vi "create_marker_channel.vi"(10 "Data from Stream":cluster{"LED1?":bool, "Data":dbl}[](array[cluster])) -> (1 "LED1?":waveform(dbl), 2 "Signal":waveform(dbl))   [LabVIEW 2014]
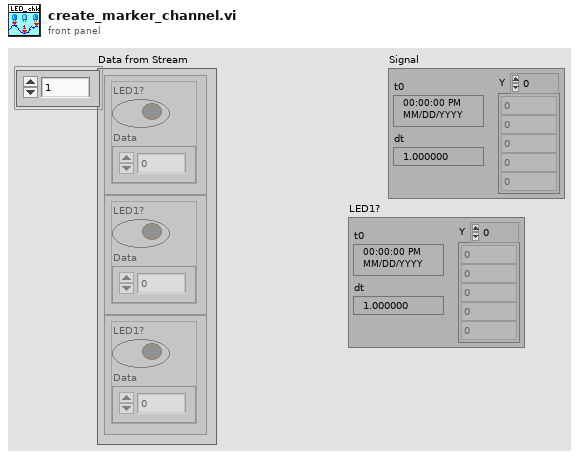
[diagram p1: front panel]
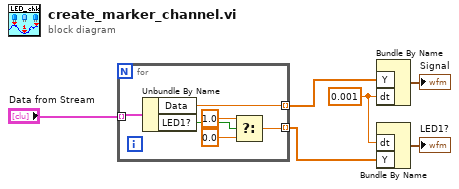
[diagram p0: block diagram]
diagram:
  w3 = 0.001 ("dt")
  n1 = for {
    tunnel: "Data from Stream" -> [w12] mode=indexing
    tunnel: [w11] -> w5 mode=indexing
    tunnel: [w7] -> w2 mode=indexing
    n2 = Unbundle By Name(w12) -> ("Data"=w11:dbl, "LED1?"=w10:bool)
    n3 = Select(t=1.0, s=w10, f=0.0) -> (s? t:f=w7:dbl)
  }
  n4 = Bundle By Name("Y"=w5, "dt"=w3) -> (→"Signal":waveform(dbl))  [unwired: 1 in]
  n5 = Bundle By Name("dt"=w3, "Y"=w2) -> (→"LED1?":waveform(dbl))  [unwired: 1 in]
